vi "Init with SQL Record.vi"(8 "error in (no error)":errorcluster, 10 "MySQL Record":variant[](array[variant]), 11 "Transaction in":refnum<class "Transaction.lvclass">) -> (0 "error out":errorcluster, 3 "Transaction out":refnum<class "Transaction.lvclass">)   [LabVIEW 2018, in "Transaction.lvclass"]
uses:
  Transaction.lvclass
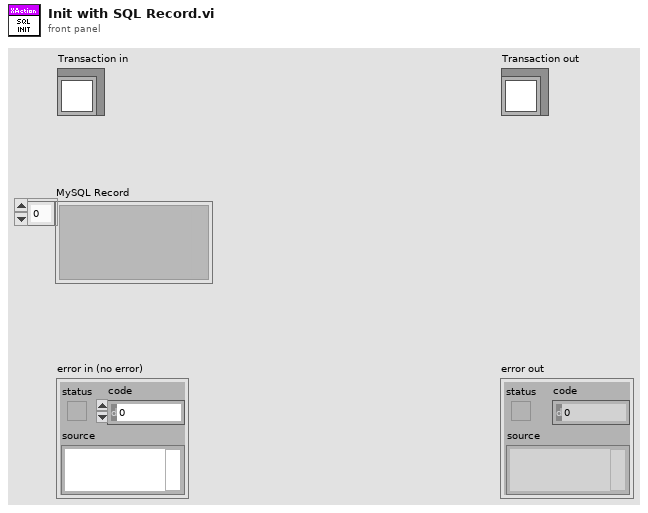
[diagram p1: front panel]
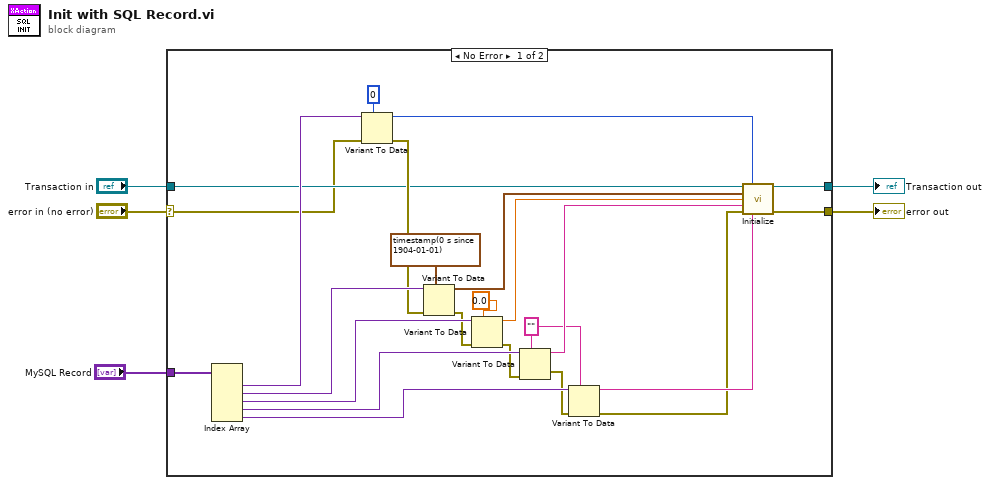
[diagram p0: block diagram]
diagram:
  n1 = case shown="No Error" "error in (no error)" {
    selector: "error in (no error)" -> [w7 w30]
    tunnel: [w8 w31] -> w3
    tunnel: "Transaction in" -> [w9 w31]
    tunnel: "MySQL Record" -> [w10 _]
    tunnel: [w6 w30] -> w1
    frame No Error {
      w13 = ""
      n2 = Index Array(array=w10) -> (element #1=w19:variant, element #2=w23:variant, element #3=w20:variant, element #4=w21:variant, element #5=w22:variant)  [unwired: 5 in]
      n3 = Variant To Data(error in=w7, type=0 ("id"), Variant=w19) -> (data=w24:i32, error out=w15:errorcluster)
      n4 = Variant To Data(error in=w15, type=timestamp(0 s since 1904-01-01), Variant=w23) -> (data=w25:timestamp, error out=w18:errorcluster)
      n5 = Variant To Data(error in=w18, type=0.0 ("Amount"), Variant=w20) -> (data=w27:dbl, error out=w17:errorcluster)
      n6 = Variant To Data(error in=w17, type=w13, Variant=w21) -> (data=w28:string, error out=w16:errorcluster)
      n7 = Variant To Data(error in=w16, type=w13, Variant=w22) -> (data=w29:string, error out=w26:errorcluster)
      n8 = call "Initialize.vi"("Transaction in"=w9, "ID"=w24, "Date"=w25, "Amount"=w27, "Description"=w28, "error in (no error)"=w26, "Category"=w29) -> ("Transaction out"=w8:refnum<class "Transaction.lvclass">, "error out"=w6:errorcluster)  [unwired: 7 in]
    }
    frame Error {
    }
  }
  "error out" <- w1
  "Transaction out" <- w3
